vi "AuMT8852B SCO Loopback Mode.vi"(5 "Loopback? (T)":bool, 7 "Set/Get (Set)":enum16{"Set", "Get"}(ring), 8 "error in (no error)":errorcluster, 11 "VISA session":refnum<visa-resource-name>) -> (0 "error out":errorcluster, 2 "error code":i32, 3 "VISA session out":refnum<visa-resource-name>, 4 "Loopback? out":bool)   [LabVIEW 2017]
doc: "Anritsu MT8852B Bluetooth Tester\n\nThis command is used to set the unit into remote loopback mode. In this mode all data received over air (including SCO data) will be looped back and sent back out over air. \nThe command is only allowed when there is an ACL connection but no SCO connection. \n\nINPUTS\nSet/Get - whether the value is being sent to or retrieved from the instrument.\nLoopback? - whether to turn loopback mode on or off.\n\nOUTPUTS\nLoopback? out - whether or not loopback mode is currently enabled."
uses:
  <instrlib>/aumt8852B/General/Utilities/MT8850 Attribute ID.ctl
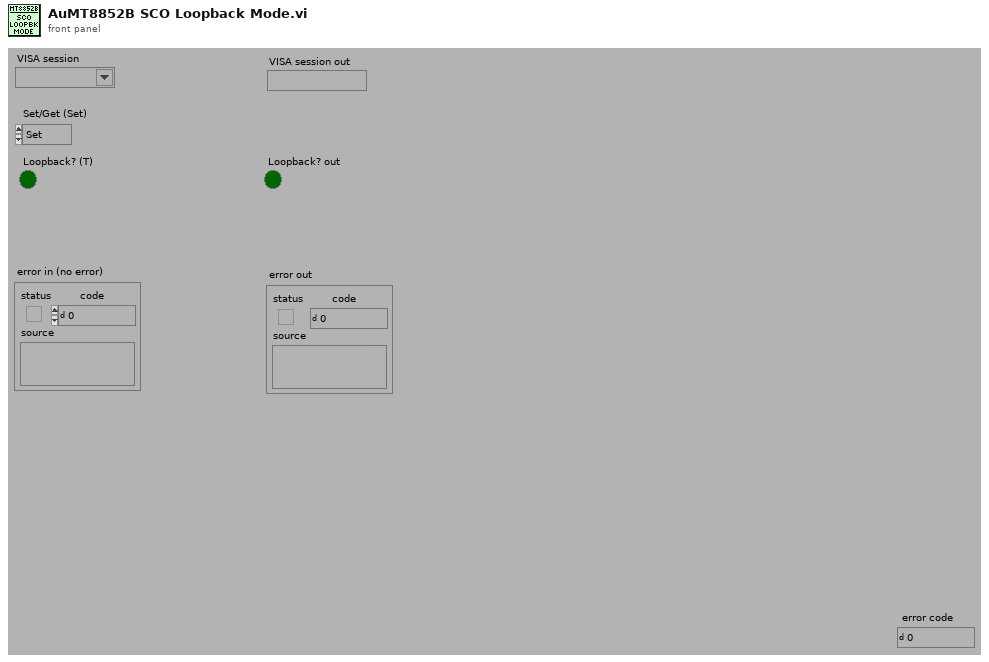
[diagram p1: front panel]
types:
  T1 = typedef "MT8850 Attribute ID.ctl" = enum16{"Operation mode", "Selected script", "EUT address source", "EUT Address", "EUT HCI RS232 Baud Rate", "Tester GPIB Address", "Tester RS232 Baud Rate", "Tester Bluetooth Address", "Tester Contrast", "Tester Key Click On", "Tester Modulation Index", "Tester Poll-Null Mode", "Tester Power Range", "Tester RS232 Mode", "Beep on Illegal Entry", "Display User Text", "User Text", "Calibration TX Modulation DAC", "Calibration RX Channel", "Calibration TX Channel", "Calibration TX Power", "Calibration Use TX Table", "Inquiry Request User-friendly Name", "Inquiry Number of Responses", "Inquiry Timeout", "Script Frequency Display", "Script Loop Count", "Script Loop Continuously", "Script Loop Stop on Fail", "Link timeout", "Page timeout", "Filter bandwidth", "SCO air code", "SCO bit position", "SCO input code", "SCO input data", "SCO input sample size", "SCO loopback mode", "SCO packet type", "SCO tone generator", "Tester page scan repetition mode", "Tester follow test mode", "Tester authentication state", "Tester authentication pin code", "Tester authentication pin length"}
  T2 = typedef "Attribute Status.ctl" = enum16{"No I/O needed", "I/O needed"}
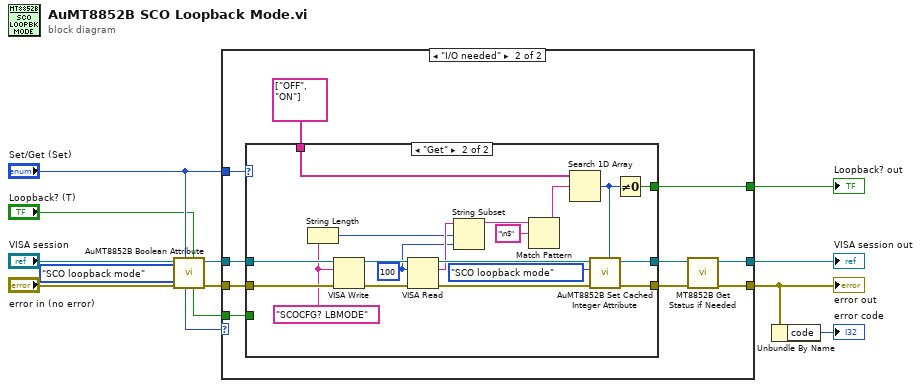
[diagram p0: block diagram]
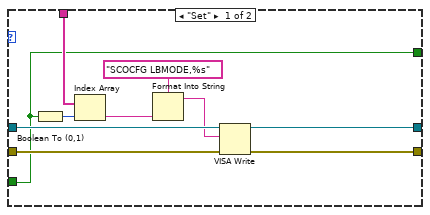
[diagram p3: hidden frame]
diagram:
  n1 = call <instrlib>:"AuMT8852B Boolean Attribute.vi"("Value (F)"="Loopback? (T)", "Set/Get (Set)"="Set/Get (Set)", "error in (no error)"="error in (no error)", "Attribute ID"=MT8850_Attribute_ID."SCO loopback mode", "VISA session"="VISA session") -> ("error out"=w10:errorcluster, "VISA session out"=w11:refnum<visa-resource-name>, "Value out"=w5:bool, "Status"=w9:T2)  [unwired: 3 in]
  n2 = case shown="\"I/O needed\"" w9 {
    tunnel: "Set/Get (Set)" -> [_ w26]
    tunnel: w5 -> [w14 w25]
    tunnel: [w15 w19] -> w1
    tunnel: [w16 w20] -> w12
    tunnel: w11 -> [w16 w24]
    tunnel: w10 -> [w15 w23]
    tunnel: [w14 w17] -> w4
    frame "No I/O needed", Default {
    }
    frame "I/O needed" {
      n3 = case shown="\"Get\"" w26 {
        tunnel: [w33 w48] -> w21
        tunnel: w25 -> [w27 _]
        tunnel: [w34 w49] -> w22
        tunnel: w24 -> [w36 w55]
        tunnel: w23 -> [w35 w54]
        tunnel: [w27 w44] -> w17
        tunnel: string[] ["OFF", "ON"] ("Array Constant") -> [w30 w45]
        frame "Set" {
          n4 = Boolean To (0,1)(Boolean=w27) -> (0, 1=w28:i16)
          n5 = Index Array(array=w30, index=w28) -> (element=w29:string)
          n6 = Format Into String(format string="SCOCFG LBMODE,%s" ("Format String"), w29) -> (resulting string=w31:string)  [unwired: 2 in, 1 out]
          n7 = VISA Write(VISA resource name=w36, write buffer=w31, error in (no error)=w35) -> (VISA resource name out=w34:refnum<visa-resource-name>, error out=w33:errorcluster)  [unwired: 1 out]
        }
        frame "Get" {
          w37 = u32 100 ("byte count (0)")
          w42 = "SCOCFG? LBMODE" ("write buffer (\"\")")
          n8 = String Length(string=w42) -> (length=w41:i32)
          n9 = VISA Write(VISA resource name=w55, write buffer=w42, error in (no error)=w54) -> (VISA resource name out=w53:refnum<visa-resource-name>, error out=w52:errorcluster)  [unwired: 1 out]
          n10 = VISA Read(VISA resource name=w53, byte count=w37, error in (no error)=w52) -> (VISA resource name out=w51:refnum<visa-resource-name>, read buffer=w46:string, error out=w50:errorcluster)  [unwired: 1 out]
          n11 = String Subset(string=w46, offset (0)=w41, length (rest)=w37) -> (substring=w40:string)
          n12 = Match Pattern(string=w40, regular expression="\n$") -> (before substring=w39:string)  [unwired: 1 in, 3 out]
          n13 = Search 1D Array(1D array=w45, element=w39) -> (index of element=w43:i32)  [unwired: 1 in]
          n14 = call <instrlib>:"AuMT8852B Set Cached Integer Attribute.vi"("Value (0)"=w43, "error in (no error)"=w50, "Attribute ID"=MT8850_Attribute_ID."SCO loopback mode", "VISA session"=w51) -> ("error out"=w48:errorcluster, "VISA session out"=w49:refnum<visa-resource-name>)  [unwired: 6 in]
          n15 = Not Equal To 0?(x=w43) -> (x != 0?=w44:bool)
        }
      }
      n16 = call <instrlib>:"MT8852B Get Status if Needed.vi"("error in (no error)"=w21, "VISA session"=w22) -> ("error out"=w19:errorcluster, "VISA session out"=w20:refnum<visa-resource-name>)  [unwired: 8 in]
    }
  }
  "error out" <- w1
  "VISA session out" <- w12
  "Loopback? out" <- w4
  n17 = Unbundle By Name(w1) -> ("code"=→"error code":i32)
